vi "#24.vi"(0 "System no.":i32=1 min=1 max=4 step=1, 5 "error in":errorcluster) -> (19 "error out":errorcluster)   [LabVIEW 2026]
doc: "Stops all motion (by sending the single ASCII character 24). #24 sets error code 10, call ERR?.vi to reset error after #24 has been called.\n\nValid for Analog systems, C-413, C-702, C-843, C-843.PM, C-844, C-848, C-865, C-866, C-867, C-877, C-880, C-880K005, C-884, C-885, C-886, C-887, C-891, E-135, E-516, E-517, E-518, E-709, E-712, E-725, E-727, E-753, E-754, E-755, E-761, E-816, E-861, E-870, E-871, E-872, E-873, E-874, F-206, Hydra, Pollux, M-8X0, Mercury, Mercury_GCS (but must be present for E-710 also). To support analog interfacing, VI must be present for E-816 also.\n\nAnalog systems: #24 does not set any error code. When used with any digital controller, does not influence connection between selected analog input channel and axis.\n\nC-880K005: VI only supported when called through PI_Multix.vi\n\nE-761: #24 does not take effect to analog input which is used for \"direct\" axis control (see the E-761 User manual). To disable \"direct\" control for an axis, the value of the corresponding \"Aux-Input to target factor\" parameter (ID 0x06000902) must be set to 0 with SPA.\n\nE-816: This command cannot be issued to a slave. Check controller manual to find out if #24 is supported.\n\nC-887, F-206, M-8X0: Depending on the firmware version on the controller, this command may not take immediate effect for motion initiated by INI or fast scanning commands."
panel:
  # "Sends ASCII #24 without LineFeed, stops motion or fast scan routines."
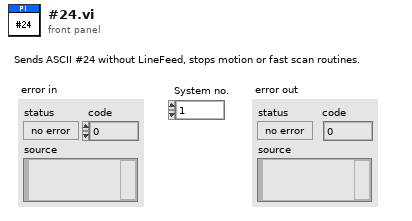
[diagram p1: front panel]
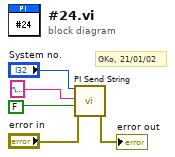
[diagram p0: block diagram]
diagram:
  # "GKo, 21/01/02"
  n1 = call "PI Send String.vi"("System no."="System no.", "String to send"="\u0018", "Attach termination char.?"=FALSE ("Attach Linefeed?"), "error in"="error in") -> ("error out"=→"error out":errorcluster)  [unwired: 15 out]
